vi "CheckReadyToSend.vi"(10 "data in progress":variant, 11 "online":bool) -> (3 "read to send":bool)   [LabVIEW 2017, in "FileManager.lvlib"]
uses:
  <vilib>/addons/InsightCM/Devices/Shared/Common/FileManager/FileManager.lvlib
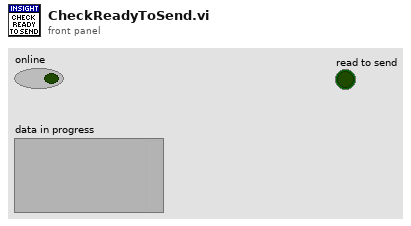
[diagram p1: front panel]
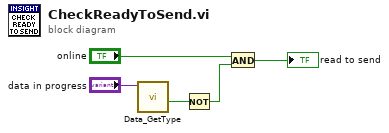
[diagram p0: block diagram]
diagram:
  n1 = call <vilib>:"Data_GetType.vi"("data"="data in progress") -> ("in progress"=w1:bool)  [unwired: 7 in, 3 out]
  n2 = Not(x=w1) -> (.not. x?=w5:bool)
  n3 = And(x="online", y=w5) -> (x .and. y?=→"read to send":bool)
